vi "Finalize To Settings.vi"(8 "error in":errorcluster, 11 "RDMA Rx Transfer Configuration in":refnum<class "RDMA Transfer Rx Configuration.lvclass">=refnum) -> (0 "error out":errorcluster, 2 "settings":cluster{"key":string, "value":string}[](array[cluster]), 3 "RDMA Rx Transfer Configuration out":refnum<class "RDMA Transfer Rx Configuration.lvclass">)   [LabVIEW 2020, in "RDMA.lvlib" / "RDMA Transfer Rx Configuration.lvclass"]
uses:
  RDMA Transfer Rx Configuration.lvclass
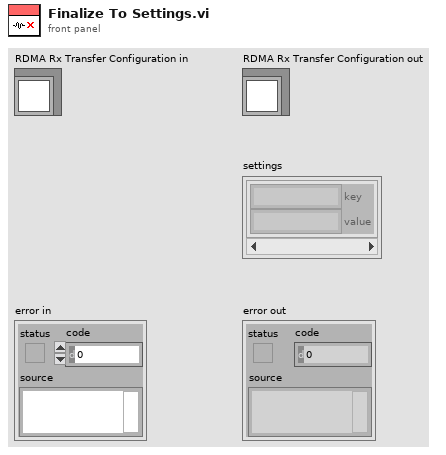
[diagram p1: front panel]
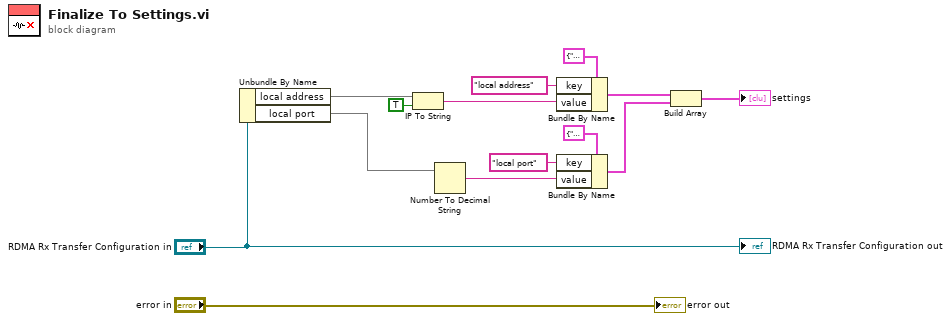
[diagram p0: block diagram]
diagram:
  n1 = Unbundle By Name("RDMA Rx Transfer Configuration in") -> ("local address"=w10, "local port"=w5)
  n2 = IP To String(1:TRUE ("dot notation? (F)"), 2:w10) -> (0:w8:string)
  n3 = Number To Decimal String(number=w5) -> (decimal integer string=w4:string)  [unwired: 1 in]
  n4 = Bundle By Name(cluster=cluster{"key":string, "value":string} {"key"="", "value"=""} ("setting"), "key"="local address", "value"=w8) -> (w3:cluster{"key":string, "value":string})
  n5 = Bundle By Name(cluster=cluster{"key":string, "value":string} {"key"="", "value"=""} ("setting"), "key"="local port", "value"=w4) -> (w2:cluster{"key":string, "value":string})
  n6 = Build Array(w3, w2) -> (→"settings":cluster{"key":string, "value":string}[])
  "error out" <- "error in"
  "RDMA Rx Transfer Configuration out" <- "RDMA Rx Transfer Configuration in"
